vi "SDCP BTR Decode.vi"(2 "error in (no error)":errorcluster, 3 "Frame":u8[](array[numeric]), 4 "in":T1) -> (0 "error out":errorcluster, 1 "out":T1)   [LabVIEW 2020]
uses:
  Typedefs/SDCP BTR Params.ctl
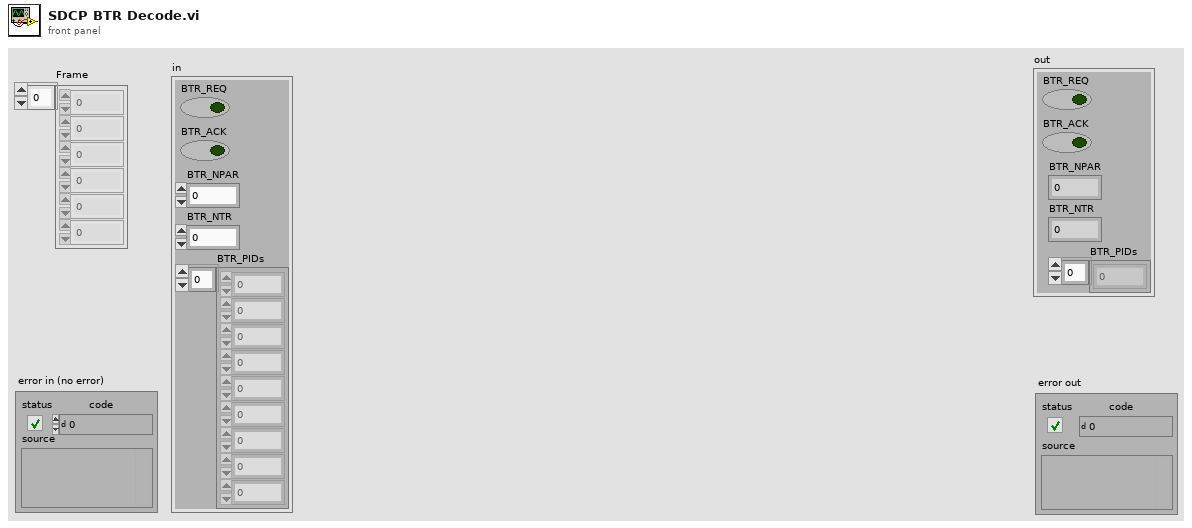
[diagram p1: front panel]
types:
  T1 = typedef "SDCP BTR Params.ctl" = cluster{"BTR_REQ":bool, "BTR_ACK":bool, "BTR_NPAR":i32, "BTR_NTR":i32, "BTR_PIDs":u8[]}
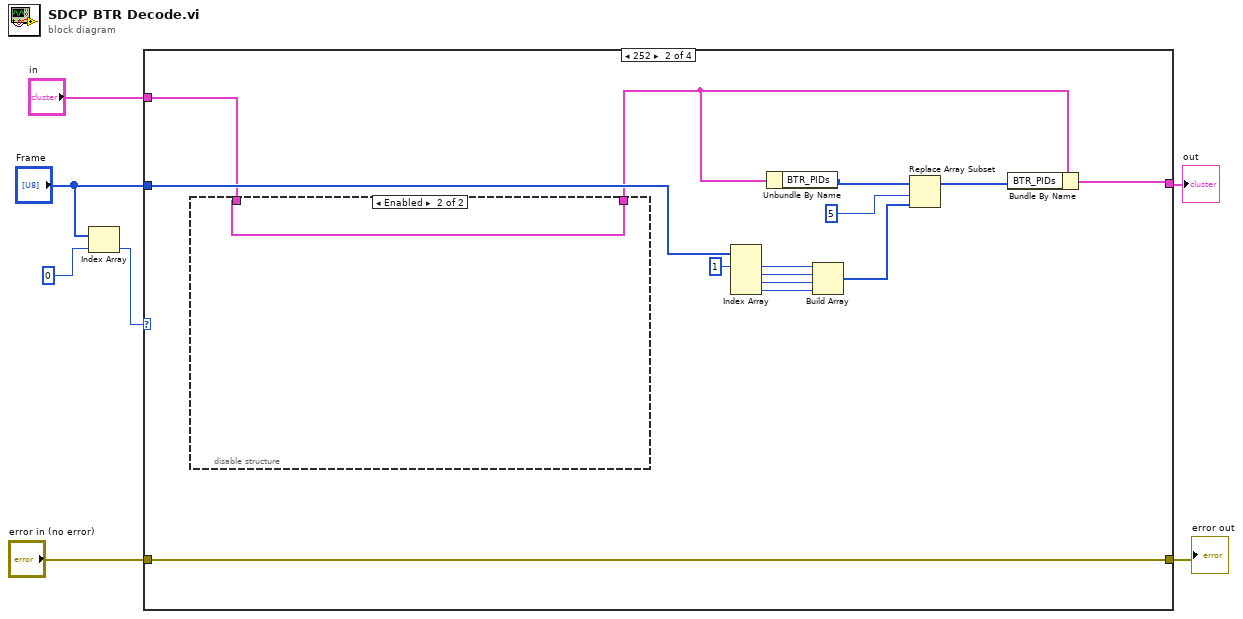
[diagram p0: block diagram]
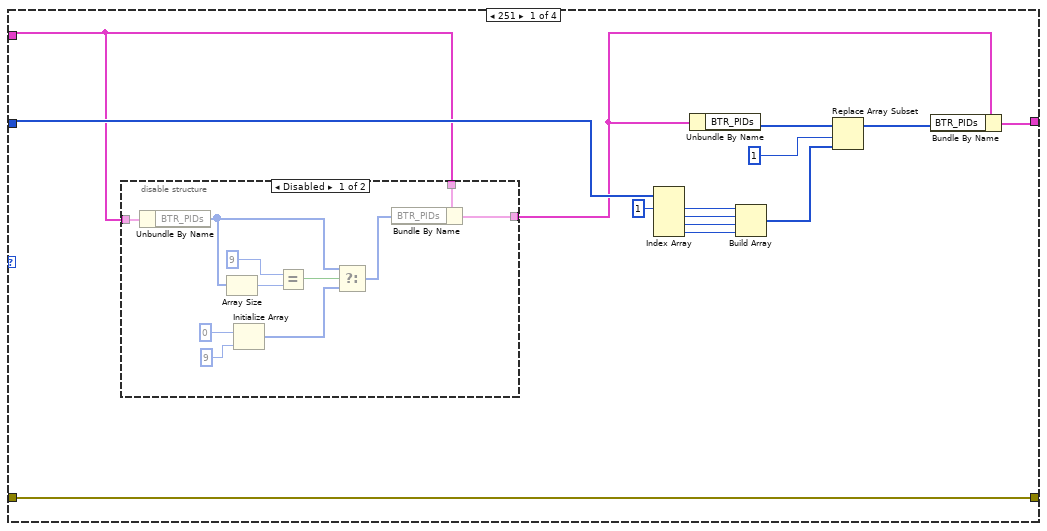
[diagram p2: hidden frame]
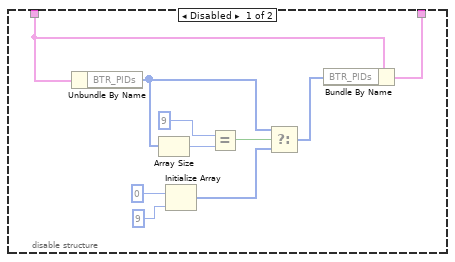
[diagram p4: hidden frame]
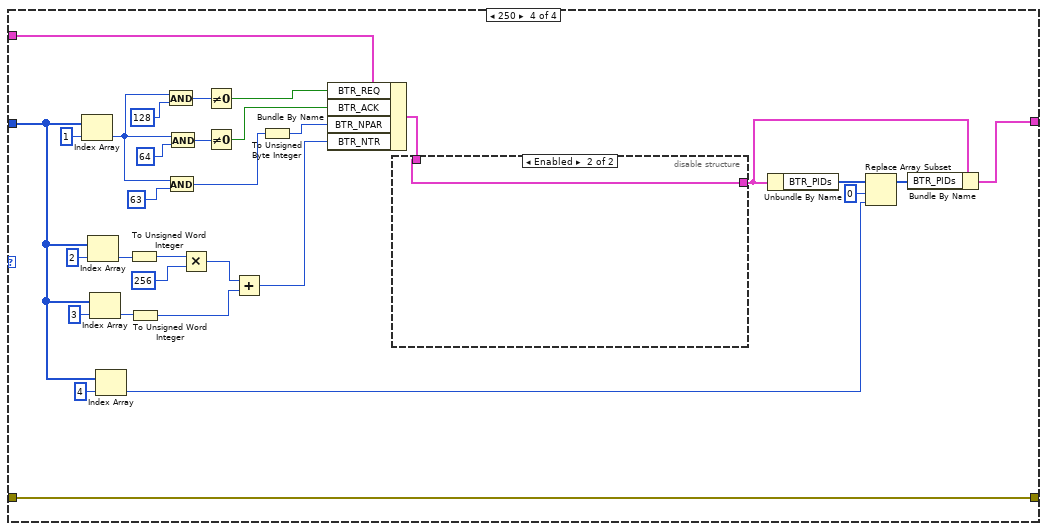
[diagram p6: hidden frame]
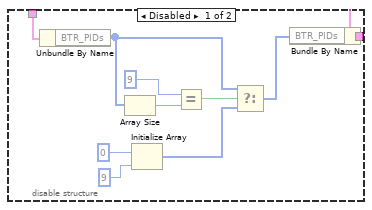
[diagram p7: hidden frame]
diagram:
  n1 = Index Array(array="Frame", index=0) -> (element=w3:u8)
  n2 = case shown="252" w3 {
    tunnel: "error in (no error)" -> [w21 w47 w60 w91]
    tunnel: [w21 w47 w60 w91] -> w5
    tunnel: "in" -> [w8 w35 w59 w83]
    tunnel: "Frame" -> [w20 w37 _ w67]
    tunnel: [w9 w36 w59 w63] -> w1
    frame 251 {
      n3 = disable-structure shown="Disabled" {
        disable-tunnel: w8 -> [w24 w33]
        disable-tunnel: [w23 w33] -> w10
        disable-tunnel: w8 -> [w22 _]
        frame Disabled {
          n4 = Unbundle By Name(w24) -> ("BTR_PIDs"=w29:u8[])
          n5 = Array Size(array=w29) -> (size(s)=w32:i32)
          n6 = Initialize Array(u8 0, 9 ("dimension size")) -> (w26:u8[])
          n7 = Equal?(x=9, y=w32) -> (x = y?=w30:bool)
          n8 = Select(t=w29, s=w30, f=w26) -> (s? t:f=w25:u8[])
          n9 = Bundle By Name(cluster=w22, "BTR_PIDs"=w25) -> (w23:T1)
        }
        frame Enabled {
        }
      }
      n10 = Index Array(array=w20, index #1=1 ("index")) -> (element #1=w18:u8, element #2=w17:u8, element #3=w16:u8, element #4=w15:u8)  [unwired: 3 in]
      n11 = Unbundle By Name(w10) -> ("BTR_PIDs"=w11:u8[])
      n12 = Build Array(w18, w17, w16, w15) -> (w14:u8[])
      n13 = Replace Array Subset(array=w11, new element=w14, index=1) -> (w12:u8[])
      n14 = Bundle By Name(cluster=w10, "BTR_PIDs"=w12) -> (w9:T1)
    }
    frame 252 {
      n15 = disable-structure shown="Enabled" {
        disable-tunnel: w35 -> [w49 w58]
        disable-tunnel: [w48 w58] -> w34
        frame Disabled {
          n16 = Unbundle By Name(w49) -> ("BTR_PIDs"=w54:u8[])
          n17 = Array Size(array=w54) -> (size(s)=w57:i32)
          n18 = Initialize Array(u8 0, 9 ("dimension size")) -> (w51:u8[])
          n19 = Equal?(x=9, y=w57) -> (x = y?=w55:bool)
          n20 = Select(t=w54, s=w55, f=w51) -> (s? t:f=w50:u8[])
          n21 = Bundle By Name(cluster=w49, "BTR_PIDs"=w50) -> (w48:T1)
        }
        frame Enabled {
        }
      }
      n22 = Index Array(array=w37, index #1=1 ("index")) -> (element #1=w45:u8, element #2=w44:u8, element #3=w43:u8, element #4=w42:u8)  [unwired: 3 in]
      n23 = Unbundle By Name(w34) -> ("BTR_PIDs"=w41:u8[])
      n24 = Build Array(w45, w44, w43, w42) -> (w40:u8[])
      n25 = Replace Array Subset(array=w41, new element=w40, index=5) -> (w38:u8[])
      n26 = Bundle By Name(cluster=w34, "BTR_PIDs"=w38) -> (w36:T1)
    }
    frame Default {
    }
    frame 250 {
      n27 = Index Array(array=w67, index=1) -> (element=w87:u8)
      n28 = Index Array(array=w67, index=2) -> (element=w76:u8)
      n29 = Index Array(array=w67, index=3) -> (element=w75:u8)
      n30 = Index Array(array=w67, index=4) -> (element=w65:u8)
      n31 = To Unsigned Word Integer(number=w76) -> (unsigned 16bit integer=w74:u16)
      n32 = To Unsigned Word Integer(number=w75) -> (unsigned 16bit integer=w71:u16)
      n33 = And(x=w87, y=u8 128) -> (x .and. y?=w85:u8)
      n34 = And(x=w87, y=u8 63) -> (x .and. y?=w80:u8)
      n35 = And(x=w87, y=u8 64) -> (x .and. y?=w84:u8)
      n36 = Multiply(x=w74, y=u16 256) -> (x*y=w72:u16)
      n37 = Not Equal To 0?(x=w85) -> (x != 0?=w82:bool)
      n38 = Not Equal To 0?(x=w84) -> (x != 0?=w81:bool)
      n39 = Add(x=w72, y=w71) -> (x+y=w70:u16)
      n40 = To Unsigned Byte Integer(number=w80) -> (unsigned 8bit integer=w79:u8)
      n41 = Bundle By Name(cluster=w83, "BTR_REQ"=w82, "BTR_ACK"=w81, "BTR_NPAR"=w79, "BTR_NTR"=w70) -> (w62:T1)
      n42 = disable-structure shown="Enabled" {
        disable-tunnel: w62 -> [w94 w102]
        disable-tunnel: [w93 w102] -> w61
        frame Disabled {
          n43 = Unbundle By Name(w94) -> ("BTR_PIDs"=w98:u8[])
          n44 = Array Size(array=w98) -> (size(s)=w101:i32)
          n45 = Initialize Array(u8 0, 9 ("dimension size")) -> (w95:u8[])
          n46 = Equal?(x=9, y=w101) -> (x = y?=w99:bool)
          n47 = Select(t=w98, s=w99, f=w95) -> (s? t:f=w92:u8[])
          n48 = Bundle By Name(cluster=w94, "BTR_PIDs"=w92) -> (w93:T1)
        }
        frame Enabled {
        }
      }
      n49 = Unbundle By Name(w61) -> ("BTR_PIDs"=w69:u8[])
      n50 = Replace Array Subset(array=w69, new element=w65, index=0) -> (w64:u8[])
      n51 = Bundle By Name(cluster=w61, "BTR_PIDs"=w64) -> (w63:T1)
    }
  }
  "error out" <- w5
  "out" <- w1
